vi "updateDt.vi"(8 "error in (no error)":errorcluster, 10 "dt":dbl, 11 "ScriptEvent in":refnum<class "ScriptEvent.lvclass">) -> (0 "error out":errorcluster, 2 "time":dbl, 3 "ScriptEvent out":refnum<class "ScriptEvent.lvclass">)   [LabVIEW 2011, in "Tools.lvlib" / "Scripting.lvlib" / "ScriptEvent.lvclass"]
uses:
  ScriptEvent.lvclass
  ScriptEvent.lvclass/ScriptEvent.ctl
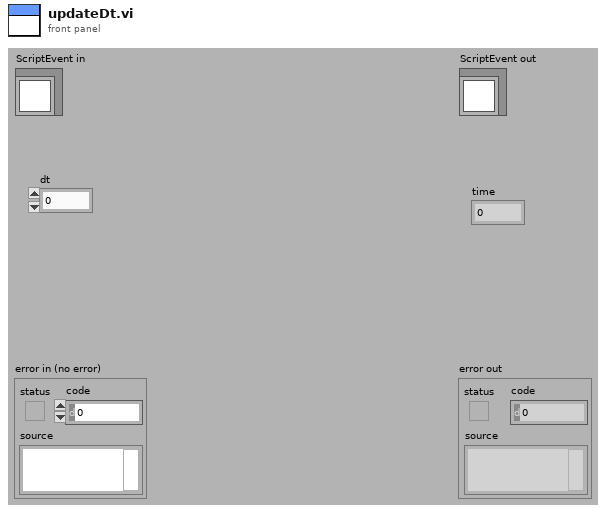
[diagram p1: front panel]
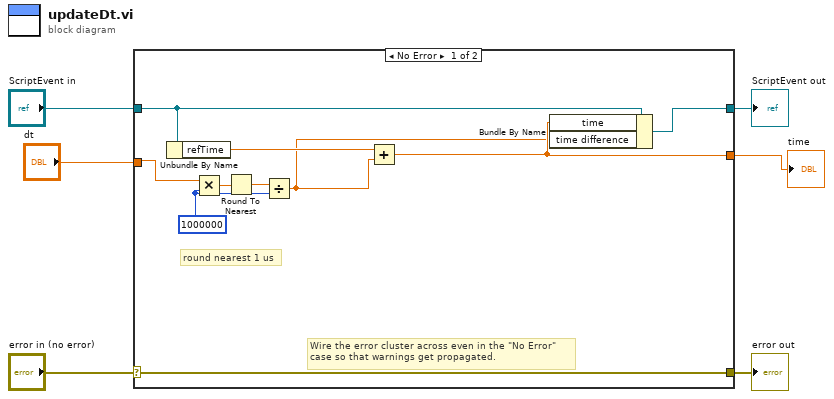
[diagram p0: block diagram]
diagram:
  n1 = case shown="No Error" "error in (no error)" {
    selector: "error in (no error)" -> [w16 w18]
    tunnel: [w16 w18] -> w5
    tunnel: [w12 w17] -> w3
    tunnel: "ScriptEvent in" -> [w13 w17]
    tunnel: "dt" -> [w8 _]
    tunnel: [w14 _] -> w1
    frame No Error {
      w9 = 1000000
      # "round nearest 1 us"
      # "Wire the error cluster across even in the \"No Error\"\ncase so that warnings get propagated."
      n2 = Unbundle By Name(w13) -> ("refTime"=w15:dbl)
      n3 = Multiply(x=w8, y=w9) -> (x*y=w11:dbl)
      n4 = Round To Nearest(number=w11) -> (nearest integer value=w10:dbl)
      n5 = Divide(x=w10, y=w9) -> (x/y=w7:dbl)
      n6 = Add(x=w15, y=w7) -> (x+y=w14:dbl)
      n7 = Bundle By Name(cluster=w13, "time"=w14, "time difference"=w7) -> (w12:refnum<class "ScriptEvent.lvclass">)
    }
    frame Error {
    }
  }
  "error out" <- w5
  "ScriptEvent out" <- w3
  "time" <- w1
